vi "lf-condition.vi"() -> ()   [LabVIEW 2019]
panel:
  in  "按键":T1
  in  "模式":T2
  in  "模式列表":T3(array[cluster])
  in  "添加设备":bool
  in  "模式":string(combo)
  out "按键编号":string
  in  "面板地址":string(combo)
  in  "按键名字":string(combo)
  in  "动作":string(combo)
  in  "模式":string(tree)
  out "node":T4(array[cluster])
  in  "停止":bool
  out "pannel-id-list":string[](array[string])
  out "Node-list":T5(array[cluster])
  in  "Node-model":T6
  in  "pannel-list":T7(array[cluster])
  in  "面板地址":string
  in  "添加面板":bool
  in  "单选按钮 2":T8(radio)
  in  "簇 6":T9
  in  "簇 5":T9
  in  "簇 4":T9
  in  "簇 3":T9
  in  "簇 2":T9
  in  "簇 1":T9
  in  "panel":string(tree)
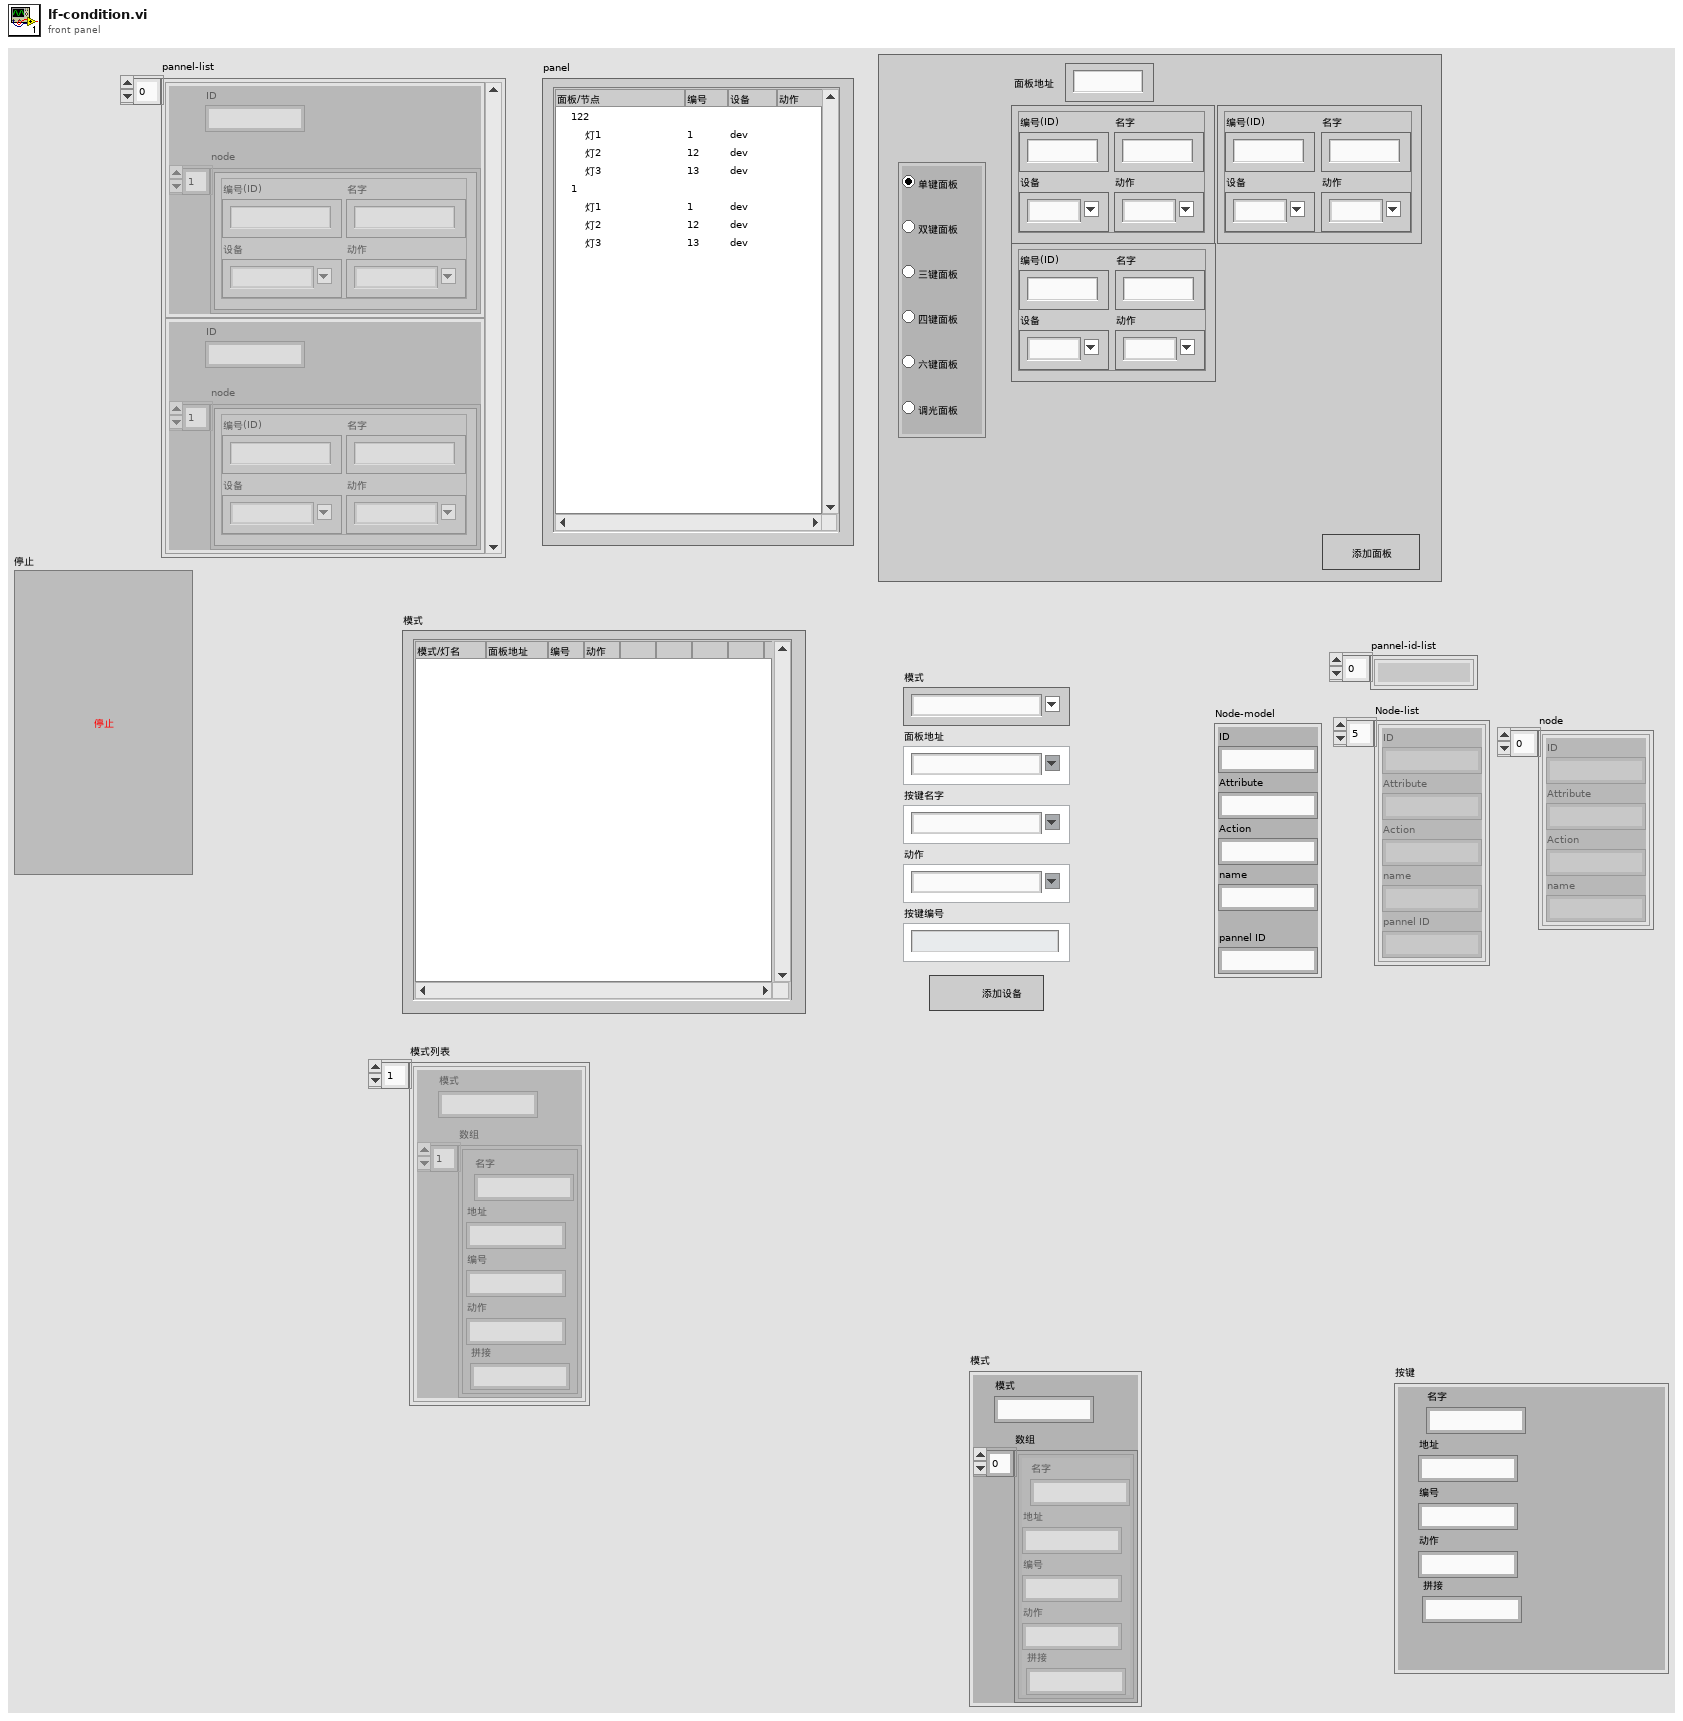
[diagram p1: front panel]
types:
  T1 = cluster{"地址":string, "名字":string, "编号":string, "动作":string, "拼接":string}
  T2 = cluster{"模式":string, "数组":cluster{"地址":string, "名字":string, "编号":string, "动作":string, "拼接":string}[]}
  T3 = cluster{"模式":string, "数组":cluster{"地址":string, "名字":string, "编号":string, "动作":string, "拼接":string}[]}[]
  T4 = cluster{"ID":string, "Attribute":string, "Action":string, "name":string}[]
  T5 = cluster{"ID":string, "Attribute":string, "Action":string, "name":string, "pannel ID":string}[]
  T6 = cluster{"ID":string, "Attribute":string, "Action":string, "name":string, "pannel ID":string}
  T7 = cluster{"node":cluster{"ID":string, "Attribute":string, "Action":string, "name":string}[], "ID":string}[]
  T8 = enum32{"单键面板", "双键面板", "三键面板", "四键面板", "六键面板", "调光面板"}
  T9 = cluster{"ID":string, "Attribute":string, "Action":string, "name":string}
  T10 = cluster{"node":cluster{"ID":string, "Attribute":string, "Action":string, "name":string}[], "ID":string}
  T11 = enum8{"Enabled", "Disabled", "Disabled and Grayed Out"}
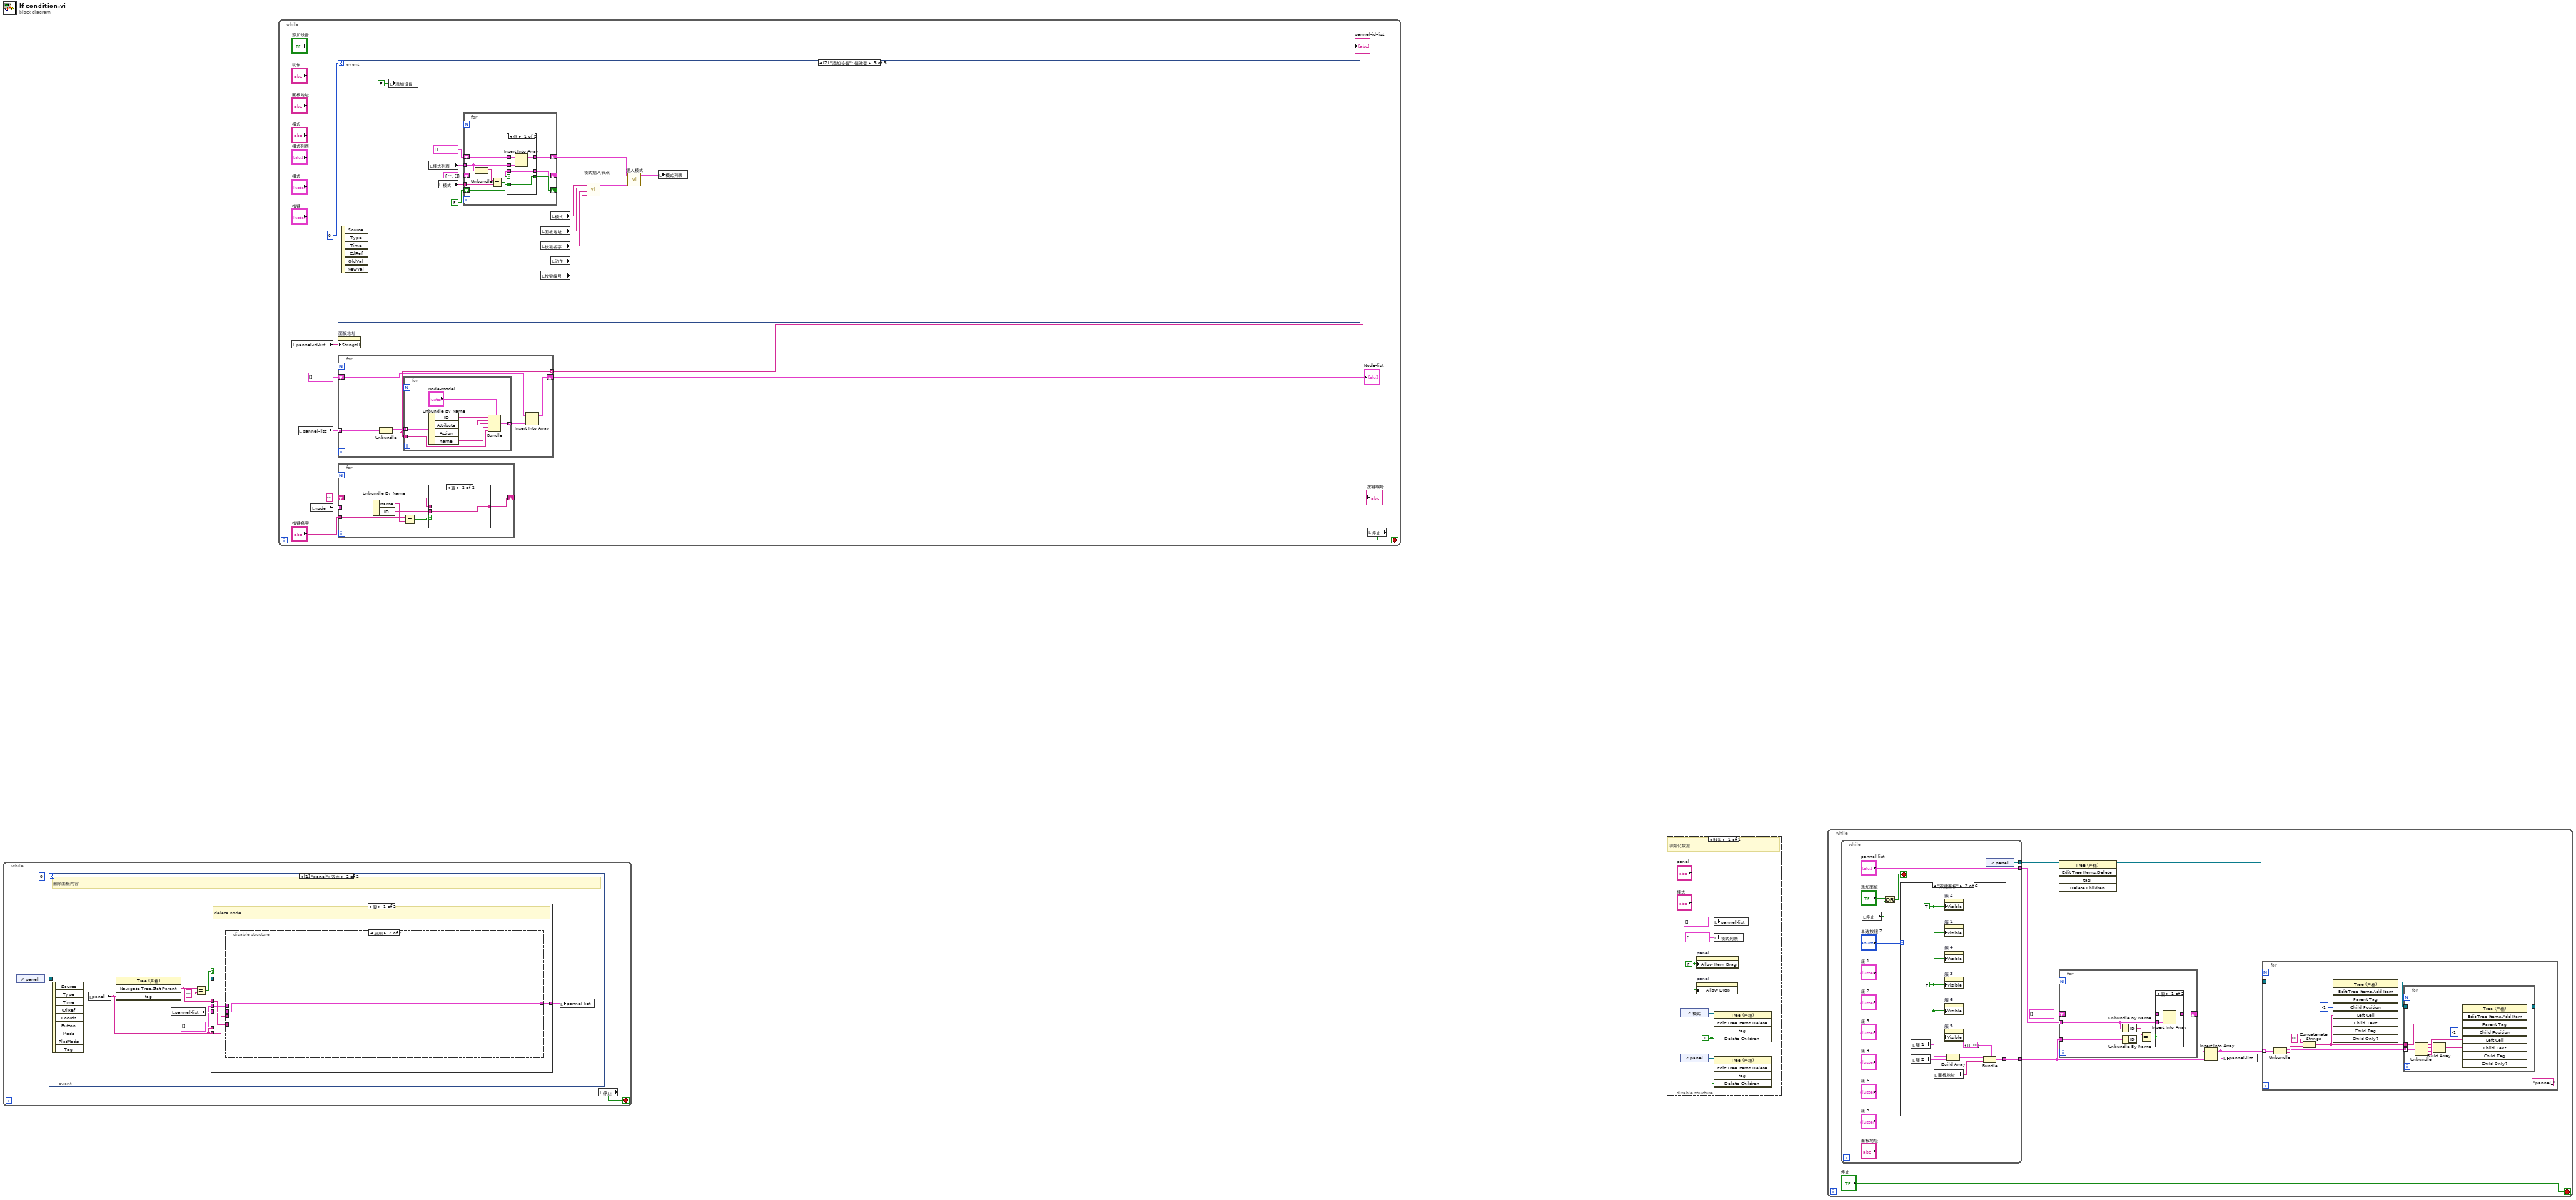
[diagram p0: block diagram]
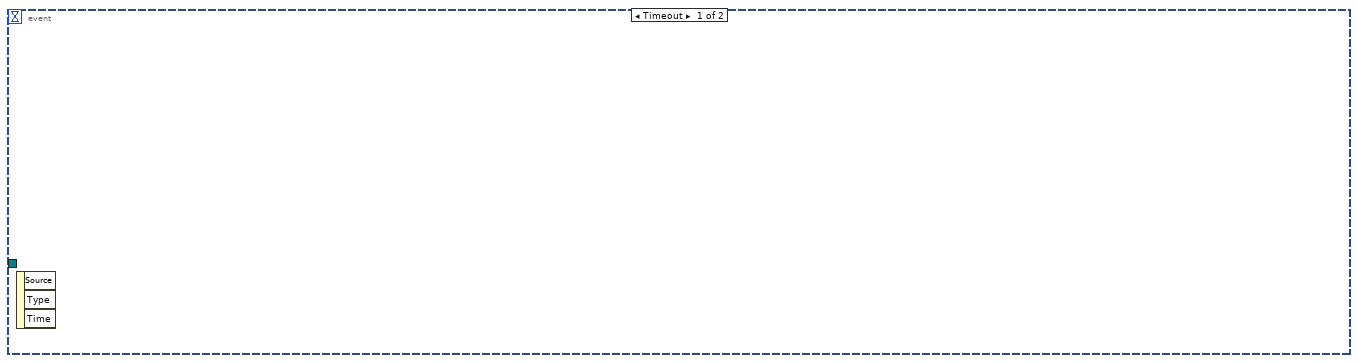
[diagram p2: hidden frame]
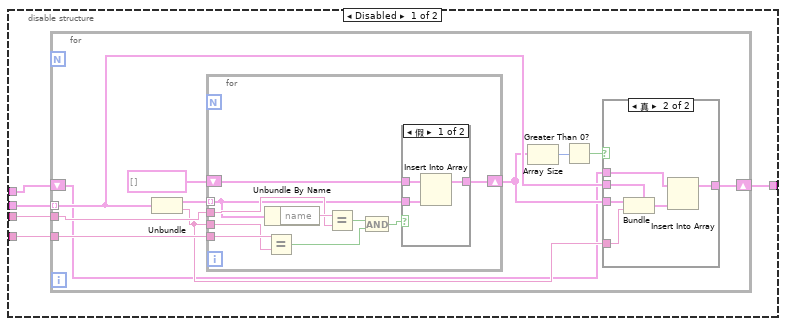
[diagram p3: hidden frame]
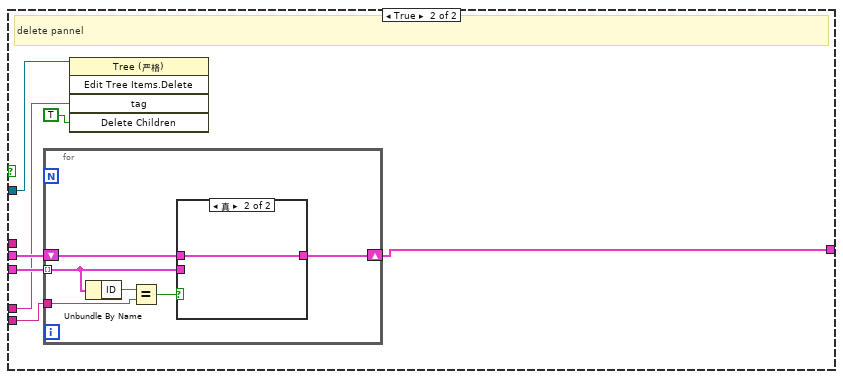
[diagram p6: hidden frame]
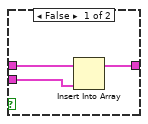
[diagram p7: hidden frame]
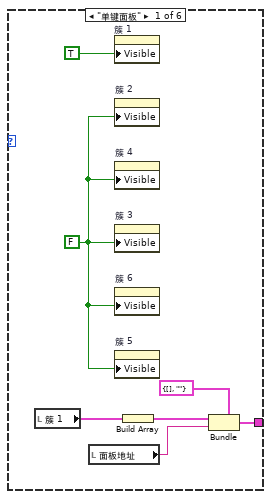
[diagram p9: hidden frame]
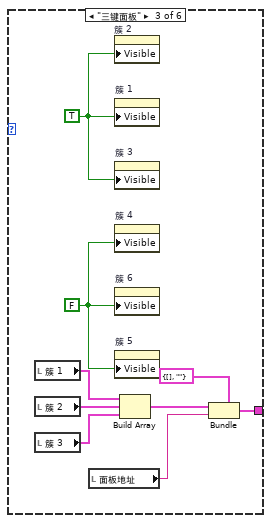
[diagram p10: hidden frame]
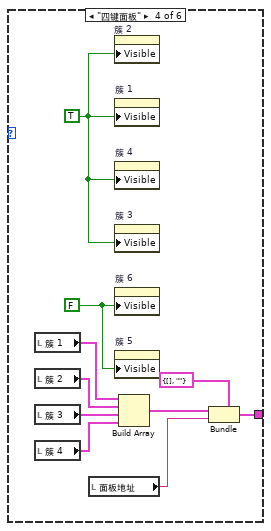
[diagram p11: hidden frame]
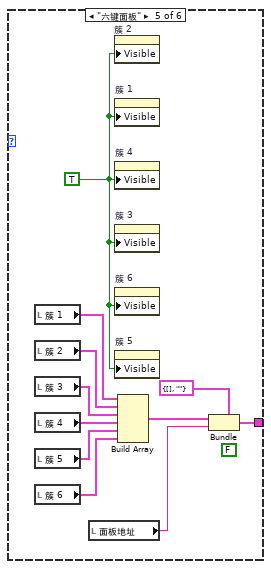
[diagram p12: hidden frame]
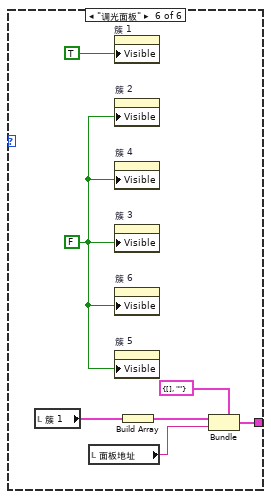
[diagram p13: hidden frame]
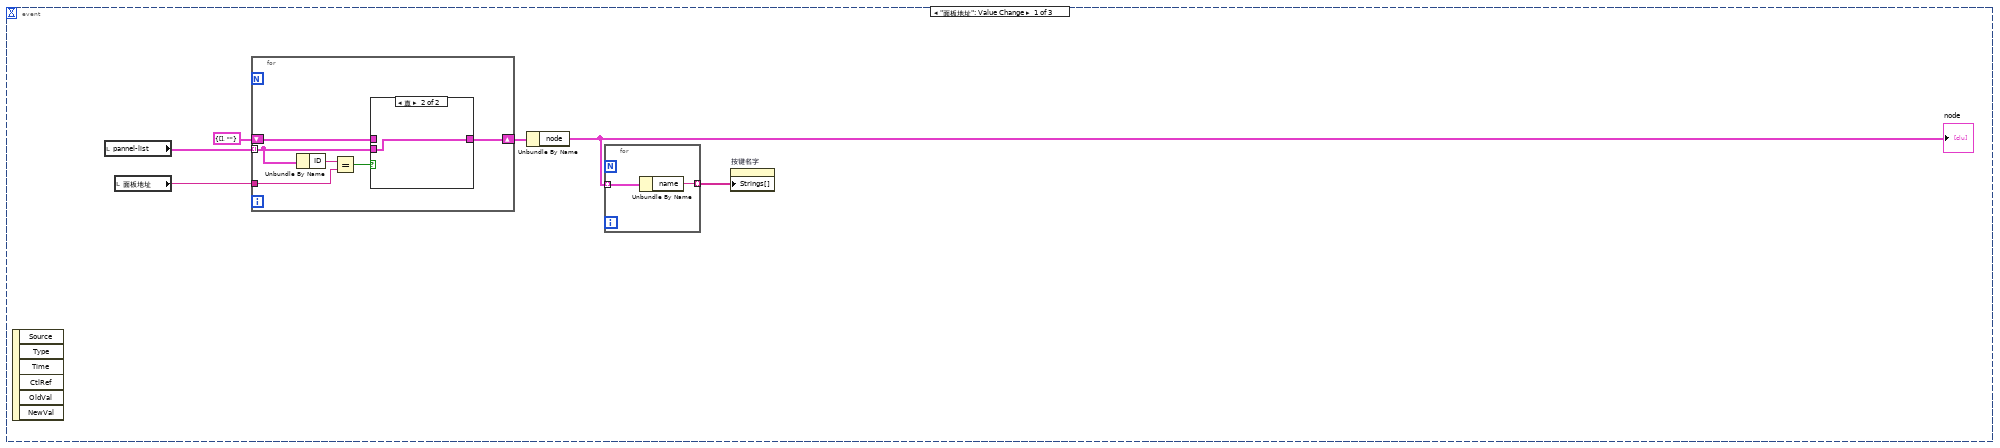
[diagram p15: hidden frame]
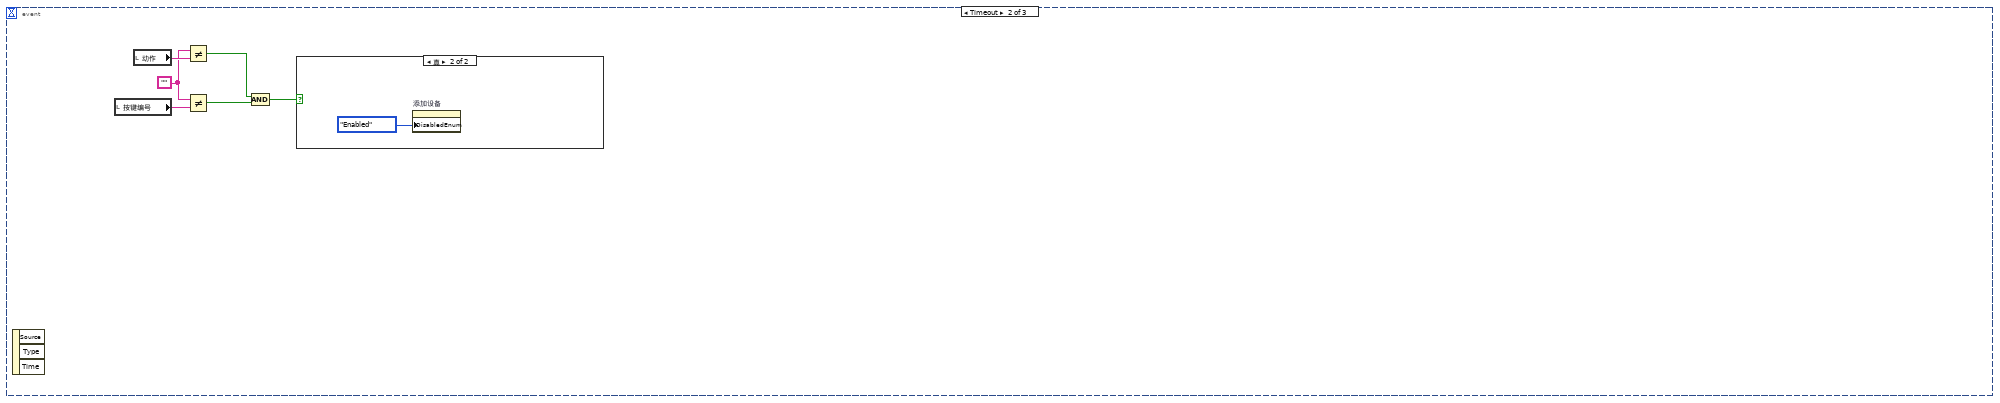
[diagram p17: hidden frame]
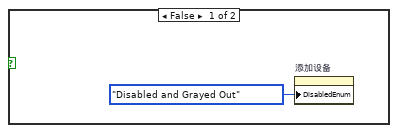
[diagram p18: hidden frame]
diagram:
  n1 = while {
    stop <- w3 stop-if-true
    n2 = control-ref of="panel"() -> (w1:refnum<vi>)
    n3 = event shown="[1] \"panel\": 双击" {
      selector: _ -> [_ _]
      dyn-events: _ -> [_ _]
      timeout: 0 -> [_ _]
      tunnel: w1 -> [_ w12]
      event Timeout {
        n4 = event-data() -> ()  [unwired: 1 in, 3 out]
      }
      event "panel": Double Click {
        # "删除面板内容"
        n5 = event-data() -> ()  [unwired: 1 in, 9 out]
        n6 = local read "panel"() -> (w4:string)
        n7 = invoke class="Tree (严格)" method="Navigate Tree.Get Parent"(reference=w12, "tag"=w4) -> (reference out=w5:refnum<vi>, "Navigate Tree:Get Parent"=w9:string)  [unwired: 2 in, 2 out]
        n8 = local read "pannel-list"() -> (w8:T7)
        n9 = Equal?(x=w9, y="") -> (x = y?=w10:bool)
        n10 = case shown="假" w10 {
          tunnel: w4 -> [w15 w61]
          tunnel: w9 -> [w16 _]
          tunnel: w8 -> [w17 w62]
          tunnel: [w14 w60] -> w7
          tunnel: T7 [] -> [w13 w59]
          tunnel: w5 -> [_ w58]
          tunnel: w4 -> [_ w57]
          frame False {
            # "delete node"
            n11 = disable-structure shown="启用" {
              disable-tunnel: w17 -> [w22 w55]
              disable-tunnel: w16 -> [w21 _]
              disable-tunnel: w15 -> [w20 _]
              disable-tunnel: [w19 w55] -> w14
              disable-tunnel: w13 -> [w18 _]
              frame Disabled {
                n12 = for {
                  tunnel: w22 -> [w28] mode=indexing
                  tunnel: w21 -> [w32]
                  tunnel: w20 -> [w31]
                  shift-right: [w25] -> w19
                  shift-left: w18 -> [w24]
                  n13 = Unbundle(w28) -> ("node"=w33:T4, "ID"=w26:string)
                  n14 = for {
                    tunnel: w33 -> [w41] mode=indexing
                    tunnel: w26 -> [w49]
                    tunnel: w32 -> [w50]
                    tunnel: w31 -> [w47]
                    shift-right: [w42] -> w27
                    shift-left: T4 [] -> [w43]
                    n15 = Unbundle By Name(w41) -> ("name"=w48:string)
                    n16 = Equal?(x=w50, y=w49) -> (x = y?=w45:bool)
                    n17 = Equal?(x=w48, y=w47) -> (x = y?=w46:bool)
                    n18 = And(x=w46, y=w45) -> (x .and. y?=w44:bool)
                    n19 = case shown="假" w44 {
                      tunnel: w43 -> [w53 w54]
                      tunnel: [w52 w54] -> w42
                      tunnel: w41 -> [w51 _]
                      frame False {
                        n20 = Insert Into Array(array=w53, new element=w51) -> (w52:T4)  [unwired: 1 in]
                      }
                      frame True {
                      }
                    }
                  }
                  n21 = Array Size(array=w27) -> (size(s)=w30:i32)
                  n22 = Greater Than 0?(x=w30) -> (x > 0?=w29:bool)
                  n23 = case shown="真" w29 {
                    tunnel: w28 -> [_ w40]
                    tunnel: w27 -> [_ w39]
                    tunnel: w26 -> [_ w38]
                    tunnel: [w34 w36] -> w25
                    tunnel: w24 -> [w34 w35]
                    frame False {
                    }
                    frame True {
                      n24 = Bundle(cluster=w40, "node"=w39, "ID"=w38) -> (w37:T10)
                      n25 = Insert Into Array(array=w35, new element=w37) -> (w36:T7)  [unwired: 1 in]
                    }
                  }
                }
              }
              frame Enabled {
              }
            }
          }
          frame True {
            # "delete pannel"
            n26 = for {
              tunnel: w62 -> [w65] mode=indexing
              tunnel: w61 -> [w67]
              shift-right: [w64] -> w60
              shift-left: w59 -> [w63]
              n27 = Unbundle By Name(w65) -> ("ID"=w68:string)
              n28 = Equal?(x=w68, y=w67) -> (x = y?=w66:bool)
              n29 = case shown="真" w66 {
                tunnel: w65 -> [w71 _]
                tunnel: [w70 w72] -> w64
                tunnel: w63 -> [w69 w72]
                frame False {
                  n30 = Insert Into Array(array=w69, new element=w71) -> (w70:T7)  [unwired: 1 in]
                }
                frame True {
                }
              }
            }
            n31 = invoke class="Tree (严格)" method="Edit Tree Items.Delete"(reference=w58, "tag"=w57, "Delete Children"=TRUE ("删除子项？")) -> ()  [unwired: 2 in, 5 out]
          }
        }
        n32 = local write "pannel-list"(w7) -> ()
      }
    }
    n33 = local read "停止"() -> (w3:bool)
  }
  n34 = while {
    stop <- w79 stop-if-true
    n35 = local read "pannel-id-list"() -> (w78:string[])
    n36 = local read "pannel-list"() -> (w80:T7)
    n37 = local read "node"() -> (w73:T4)
    n38 = event shown="[2] \"添加设备\": 值改变" {
      selector: _ -> [_ _ _]
      dyn-events: _ -> [_ _ _]
      timeout: 0 -> [_ _ _]
      event "面板地址": Value Change {
        n39 = event-data() -> ()  [unwired: 1 in, 6 out]
        n40 = local read "pannel-list"() -> (w93:T7)
        n41 = local read "面板地址"() -> (w94:string)
        n42 = for {
          tunnel: w93 -> [w103] mode=indexing
          tunnel: w94 -> [w105]
          shift-right: [w102] -> w96
          shift-left: T10 {"node"=[], "ID"=""} ("pannel") -> [w101]
          n43 = Unbundle By Name(w103) -> ("ID"=w106:string)
          n44 = Equal?(x=w106, y=w105) -> (x = y?=w104:bool)
          n45 = case shown="真" w104 {
            tunnel: w103 -> [_ w108]
            tunnel: [w107 w108] -> w102
            tunnel: w101 -> [w107 _]
            frame False {
            }
            frame True {
            }
          }
        }
        n46 = Unbundle By Name(w96) -> ("node"=w95:T4)
        "node" <- w95
        n47 = for {
          tunnel: w95 -> [w100] mode=indexing
          tunnel: [w99] -> w97 mode=indexing
          n48 = Unbundle By Name(w100) -> ("name"=w99:string)
        }
        n49 = property on="按键名字" class="CmbBox"("Strings[]"=w97) -> ()  [unwired: 2 in, 2 out]
      }
      event Timeout {
        w109 = ""
        n50 = event-data() -> ()  [unwired: 1 in, 3 out]
        n51 = local read "按键编号"() -> (w113:string)
        n52 = local read "动作"() -> (w114:string)
        n53 = Not Equal?(x=w109, y=w114) -> (x != y?=w111:bool)
        n54 = Not Equal?(x=w109, y=w113) -> (x != y?=w110:bool)
        n55 = And(x=w111, y=w110) -> (x .and. y?=w112:bool)
        n56 = case shown="真" w112 {
          frame False {
            n57 = property on="添加设备" class="Bool (严格)"("DisabledEnum"=T11."Disabled and Grayed Out" ("禁用")) -> ()  [unwired: 2 in, 2 out]
          }
          frame True {
            n58 = property on="添加设备" class="Bool (严格)"("DisabledEnum"=T11."Enabled" ("禁用")) -> ()  [unwired: 2 in, 2 out]
          }
        }
      }
      event "添加设备": Value Change {
        n59 = event-data() -> ()  [unwired: 1 in, 6 out]
        n60 = local write "添加设备"(FALSE ("添加设备")) -> ()
        n61 = local read "模式列表"() -> (w131:T3)
        n62 = local read "模式"() -> (w130:string)
        n63 = for {
          tunnel: w131 -> [w136] mode=indexing
          tunnel: w130 -> [w140]
          shift-right: [w138] -> _
          shift-left: FALSE -> [w137]
          shift-right: [w135] -> w119
          shift-left: T3 [] -> [w134]
          shift-right: [w133] -> w120
          shift-left: T2 {"模式"="", "数组"=[]} ("模式") -> [w132]
          n64 = Unbundle(w136) -> ("模式"=w141:string)  [unwired: 1 out]
          n65 = Equal?(x=w141, y=w140) -> (x = y?=w139:bool)
          n66 = case shown="假" w139 {
            selector: w139 -> [_ w149]
            tunnel: [w146 w149] -> w138
            tunnel: w137 -> [w146 _]
            tunnel: w136 -> [w145 w147]
            tunnel: [w144 w148] -> w135
            tunnel: w134 -> [w143 w148]
            tunnel: [w142 w147] -> w133
            tunnel: w132 -> [w142 _]
            frame False {
              n67 = Insert Into Array(array=w143, new element=w145) -> (w144:T3)  [unwired: 1 in]
            }
            frame True {
            }
          }
        }
        n68 = local read "面板地址"() -> (w121:string)
        n69 = local read "按键名字"() -> (w122:string)
        n70 = local read "按键编号"() -> (w124:string)
        n71 = local read "模式"() -> (w125:string)
        n72 = local read "动作"() -> (w123:string)
        n73 = call "模式插入节点.vi"("按键编号"=w124, "模式input"=w120, "动作"=w123, "按键名字"=w122, "面板地址"=w121, "模式选择"=w125) -> ("模式output"=w118:T2)  [unwired: 5 in]
        n74 = call "插入模式.vi"("模式"=w118, "模式列表"=w119) -> ("模式列表-output"=w117:T3)  [unwired: 9 in]
        n75 = local write "模式列表"(w117) -> ()
      }
    }
    n76 = property on="面板地址" class="CmbBox"("Strings[]"=w78) -> ()  [unwired: 2 in, 2 out]
    n77 = for {
      tunnel: w80 -> [w155] mode=indexing
      shift-right: [w150] -> w83
      shift-left: T5 [] -> [w152]
      tunnel: [w153] -> w81 mode=indexing
      n78 = Unbundle(w155) -> ("node"=w154:T4, "ID"=w153:string)
      n79 = for {
        tunnel: w154 -> [w163] mode=indexing
        tunnel: w153 -> [w157]
        tunnel: [w156] -> w151 mode=indexing
        n80 = Unbundle By Name(w163) -> ("ID"=w161:string, "Attribute"=w160:string, "Action"=w158:string, "name"=w159:string)
        n81 = Bundle(cluster="Node-model", "ID"=w161, "Attribute"=w160, "Action"=w158, "name"=w159, "pannel ID"=w157) -> (w156:T6)
      }
      n82 = Insert Into Array(array=w152, new element=w151) -> (w150:T5)  [unwired: 1 in]
    }
    "Node-list" <- w83
    "pannel-id-list" <- w81
    n83 = for {
      tunnel: w73 -> [w90] mode=indexing
      tunnel: "按键名字" -> [w88]
      shift-right: [w86] -> w75
      shift-left: "" ("ID") -> [w84]
      n84 = Unbundle By Name(w90) -> ("name"=w89:string, "ID"=w85:string)
      n85 = Equal?(x=w88, y=w89) -> (x = y?=w87:bool)
      n86 = case shown="真" w87 {
        tunnel: [w91 w92] -> w86
        tunnel: w85 -> [_ w92]
        tunnel: w84 -> [w91 _]
        frame False {
        }
        frame True {
        }
      }
    }
    "按键编号" <- w75
    n87 = local read "停止"() -> (w79:bool)
  }
  n88 = disable-structure shown="默认" {
    frame Enabled {
      w166 = TRUE ("删除子项？")
      w169 = FALSE ("拖曳/放置:允许放置")
      # "初始化数据"
      n89 = control-ref of="模式"() -> (w167:refnum<vi>)
      n90 = control-ref of="panel"() -> (w168:refnum<vi>)
      n91 = property on="panel" class="Tree (严格)"("Allow Item Drag"=w169) -> ()  [unwired: 2 in, 2 out]
      n92 = property on="panel" class="Tree (严格)"("Allow Drop"=w169) -> ()  [unwired: 2 in, 2 out]
      n93 = local write "pannel-list"(T7 [] ("pannel-list")) -> ()
      n94 = local write "模式列表"(T3 [] ("模式列表")) -> ()
      n95 = invoke class="Tree (严格)" method="Edit Tree Items.Delete"(reference=w167, "Delete Children"=w166) -> ()  [unwired: 3 in, 5 out]
      n96 = invoke class="Tree (严格)" method="Edit Tree Items.Delete"(reference=w168, "Delete Children"=w166) -> ()  [unwired: 3 in, 5 out]
    }
  }
  n97 = while {
    stop <- "停止" stop-if-true
    n98 = while {
      tunnel: [w210] -> w172
      tunnel: [w208] -> w175
      tunnel: ["pannel-list"] -> w174
      stop <- w211 stop-if-true
      n99 = local read "停止"() -> (w209:bool)
      n100 = Or(x="添加面板", y=w209) -> (x .or. y?=w211:bool)
      n101 = case shown="\"双键面板\"" "单选按钮 2" {
        tunnel: [w214 w221 w230 w238 w248 w259] -> w210
        frame "单键面板" {
          w219 = FALSE
          n102 = local read "簇 1"() -> (w218:T9)
          n103 = local read "面板地址"() -> (w216:string)
          n104 = property on="簇 1" class="Clust (严格)"("Visible"=TRUE) -> ()  [unwired: 2 in, 2 out]
          n105 = property on="簇 2" class="Clust (严格)"("Visible"=w219) -> ()  [unwired: 2 in, 2 out]
          n106 = property on="簇 4" class="Clust (严格)"("Visible"=w219) -> ()  [unwired: 2 in, 2 out]
          n107 = property on="簇 3" class="Clust (严格)"("Visible"=w219) -> ()  [unwired: 2 in, 2 out]
          n108 = property on="簇 6" class="Clust (严格)"("Visible"=w219) -> ()  [unwired: 2 in, 2 out]
          n109 = property on="簇 5" class="Clust (严格)"("Visible"=w219) -> ()  [unwired: 2 in, 2 out]
          n110 = Build Array(w218) -> (w217:T4)
          n111 = Bundle(cluster=T10 {"node"=[], "ID"=""} ("pannel"), "node"=w217, "ID"=w216) -> (w214:T10)
        }
        frame "双键面板" {
          w228 = FALSE
          w227 = TRUE
          n112 = local read "簇 1"() -> (w226:T9)
          n113 = local read "簇 2"() -> (w225:T9)
          n114 = local read "面板地址"() -> (w222:string)
          n115 = property on="簇 2" class="Clust (严格)"("Visible"=w227) -> ()  [unwired: 2 in, 2 out]
          n116 = property on="簇 1" class="Clust (严格)"("Visible"=w227) -> ()  [unwired: 2 in, 2 out]
          n117 = property on="簇 4" class="Clust (严格)"("Visible"=w228) -> ()  [unwired: 2 in, 2 out]
          n118 = property on="簇 3" class="Clust (严格)"("Visible"=w228) -> ()  [unwired: 2 in, 2 out]
          n119 = property on="簇 6" class="Clust (严格)"("Visible"=w228) -> ()  [unwired: 2 in, 2 out]
          n120 = property on="簇 5" class="Clust (严格)"("Visible"=w228) -> ()  [unwired: 2 in, 2 out]
          n121 = Build Array(w226, w225) -> (w224:T4)
          n122 = Bundle(cluster=T10 {"node"=[], "ID"=""} ("pannel"), "node"=w224, "ID"=w222) -> (w221:T10)
        }
        frame "三键面板" {
          w237 = FALSE
          w236 = TRUE
          n123 = local read "簇 1"() -> (w235:T9)
          n124 = local read "簇 2"() -> (w234:T9)
          n125 = local read "簇 3"() -> (w229:T9)
          n126 = local read "面板地址"() -> (w231:string)
          n127 = property on="簇 2" class="Clust (严格)"("Visible"=w236) -> ()  [unwired: 2 in, 2 out]
          n128 = property on="簇 1" class="Clust (严格)"("Visible"=w236) -> ()  [unwired: 2 in, 2 out]
          n129 = property on="簇 3" class="Clust (严格)"("Visible"=w236) -> ()  [unwired: 2 in, 2 out]
          n130 = property on="簇 4" class="Clust (严格)"("Visible"=w237) -> ()  [unwired: 2 in, 2 out]
          n131 = property on="簇 6" class="Clust (严格)"("Visible"=w237) -> ()  [unwired: 2 in, 2 out]
          n132 = property on="簇 5" class="Clust (严格)"("Visible"=w237) -> ()  [unwired: 2 in, 2 out]
          n133 = Build Array(w235, w234, w229) -> (w233:T4)
          n134 = Bundle(cluster=T10 {"node"=[], "ID"=""} ("pannel"), "node"=w233, "ID"=w231) -> (w230:T10)
        }
        frame "四键面板" {
          w247 = FALSE
          w246 = TRUE
          n135 = local read "簇 1"() -> (w243:T9)
          n136 = local read "簇 2"() -> (w242:T9)
          n137 = local read "簇 3"() -> (w244:T9)
          n138 = local read "簇 4"() -> (w245:T9)
          n139 = local read "面板地址"() -> (w239:string)
          n140 = property on="簇 2" class="Clust (严格)"("Visible"=w246) -> ()  [unwired: 2 in, 2 out]
          n141 = property on="簇 1" class="Clust (严格)"("Visible"=w246) -> ()  [unwired: 2 in, 2 out]
          n142 = property on="簇 4" class="Clust (严格)"("Visible"=w246) -> ()  [unwired: 2 in, 2 out]
          n143 = property on="簇 3" class="Clust (严格)"("Visible"=w246) -> ()  [unwired: 2 in, 2 out]
          n144 = property on="簇 6" class="Clust (严格)"("Visible"=w247) -> ()  [unwired: 2 in, 2 out]
          n145 = property on="簇 5" class="Clust (严格)"("Visible"=w247) -> ()  [unwired: 2 in, 2 out]
          n146 = Build Array(w243, w242, w244, w245) -> (w241:T4)
          n147 = Bundle(cluster=T10 {"node"=[], "ID"=""} ("pannel"), "node"=w241, "ID"=w239) -> (w238:T10)
        }
        frame "六键面板" {
          (unwired) FALSE
          w258 = TRUE
          n148 = local read "簇 1"() -> (w253:T9)
          n149 = local read "簇 2"() -> (w252:T9)
          n150 = local read "簇 3"() -> (w254:T9)
          n151 = local read "簇 4"() -> (w255:T9)
          n152 = local read "簇 5"() -> (w256:T9)
          n153 = local read "簇 6"() -> (w257:T9)
          n154 = local read "面板地址"() -> (w249:string)
          n155 = property on="簇 2" class="Clust (严格)"("Visible"=w258) -> ()  [unwired: 2 in, 2 out]
          n156 = property on="簇 1" class="Clust (严格)"("Visible"=w258) -> ()  [unwired: 2 in, 2 out]
          n157 = property on="簇 4" class="Clust (严格)"("Visible"=w258) -> ()  [unwired: 2 in, 2 out]
          n158 = property on="簇 3" class="Clust (严格)"("Visible"=w258) -> ()  [unwired: 2 in, 2 out]
          n159 = property on="簇 6" class="Clust (严格)"("Visible"=w258) -> ()  [unwired: 2 in, 2 out]
          n160 = property on="簇 5" class="Clust (严格)"("Visible"=w258) -> ()  [unwired: 2 in, 2 out]
          n161 = Build Array(w253, w252, w254, w255, w256, w257) -> (w251:T4)
          n162 = Bundle(cluster=T10 {"node"=[], "ID"=""} ("pannel"), "node"=w251, "ID"=w249) -> (w248:T10)
        }
        frame "调光面板" {
          w265 = FALSE
          n163 = local read "簇 1"() -> (w263:T9)
          n164 = local read "面板地址"() -> (w260:string)
          n165 = property on="簇 1" class="Clust (严格)"("Visible"=TRUE) -> ()  [unwired: 2 in, 2 out]
          n166 = property on="簇 2" class="Clust (严格)"("Visible"=w265) -> ()  [unwired: 2 in, 2 out]
          n167 = property on="簇 4" class="Clust (严格)"("Visible"=w265) -> ()  [unwired: 2 in, 2 out]
          n168 = property on="簇 3" class="Clust (严格)"("Visible"=w265) -> ()  [unwired: 2 in, 2 out]
          n169 = property on="簇 6" class="Clust (严格)"("Visible"=w265) -> ()  [unwired: 2 in, 2 out]
          n170 = property on="簇 5" class="Clust (严格)"("Visible"=w265) -> ()  [unwired: 2 in, 2 out]
          n171 = Build Array(w263) -> (w262:T4)
          n172 = Bundle(cluster=T10 {"node"=[], "ID"=""} ("pannel"), "node"=w262, "ID"=w260) -> (w259:T10)
        }
      }
      n173 = control-ref of="panel"() -> (w208:refnum<vi>)
    }
    n174 = invoke class="Tree (严格)" method="Edit Tree Items.Delete"(reference=w175) -> (reference out=w176:refnum<vi>)  [unwired: 4 in, 4 out]
    n175 = for {
      tunnel: w172 -> [w179]
      tunnel: w174 -> [w178] mode=indexing
      shift-right: [w180] -> w173
      shift-left: T7 [] -> [w181]
      n176 = Unbundle By Name(w178) -> ("ID"=w184:string)
      n177 = Unbundle By Name(w179) -> ("ID"=w183:string)
      n178 = Equal?(x=w184, y=w183) -> (x = y?=w182:bool)
      n179 = case shown="假" w182 {
        tunnel: w181 -> [w187 w188]
        tunnel: [w186 w188] -> w180
        tunnel: w178 -> [w185 _]
        frame False {
          n180 = Insert Into Array(array=w187, new element=w185) -> (w186:T7)  [unwired: 1 in]
        }
        frame True {
        }
      }
    }
    n181 = Insert Into Array(array=w173, new element=w172) -> (w171:T7)  [unwired: 1 in]
    n182 = local write "pannel-list"(w171) -> ()
    n183 = for {
      tunnel: w171 -> [w196] mode=indexing
      tunnel: w176 -> [w190]
      (unwired) "pannel_" ("字符串")
      n184 = Unbundle(w196) -> ("node"=w193:T4, "ID"=w195:string)
      n185 = Concatenate Strings("" ("字符串"), w195) -> (w192:string)
      n186 = invoke class="Tree (严格)" method="Edit Tree Items.Add Item"(reference=w190, "Child Position"=-1 ("子项位置"), "Left Cell"=w192) -> (reference out=w191:refnum<vi>)  [unwired: 6 in, 8 out]
      n187 = for {
        tunnel: w193 -> [w204] mode=indexing
        tunnel: w191 -> [w206]
        tunnel: w192 -> [w205]
        tunnel: [w202] -> _
        n188 = Unbundle(w204) -> ("ID"=w201:string, "Attribute"=w200:string, "Action"=w199:string, "name"=w203:string)
        n189 = Build Array(w201, w200, w199) -> (w198:string[])
        n190 = invoke class="Tree (严格)" method="Edit Tree Items.Add Item"(reference=w206, "Parent Tag"=w205, "Child Position"=-1 ("子项位置"), "Left Cell"=w203, "Child Text"=w198) -> (reference out=w202:refnum<vi>)  [unwired: 4 in, 8 out]
      }
    }
  }
